vi "Global_WC_Drive_Zero_Encoders.vi"() -> ()   [LabVIEW 2017]
panel:
  in  "Zero Encoders":bool
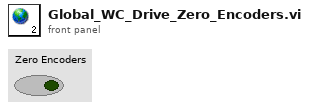
[diagram p1: front panel]
diagram:
